vi "Cool Until Target.vi"(8 "error in (no error)":errorcluster, 10 "target temperature":dbl[unit]=273.15, 11 "cooling system in":refnum<class "Cooling System.lvclass">) -> (0 "error out":errorcluster, 3 "cooling system out":refnum<class "Cooling System.lvclass">)   [LabVIEW 2023, in "Cooling System.lvclass"]
uses:
  Cooling System.lvclass
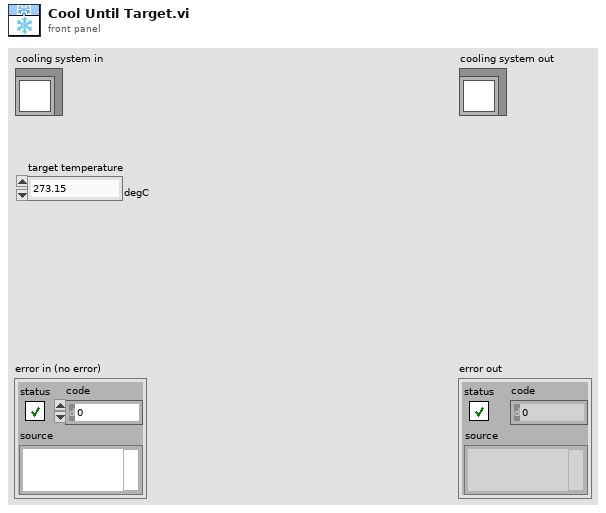
[diagram p1: front panel]
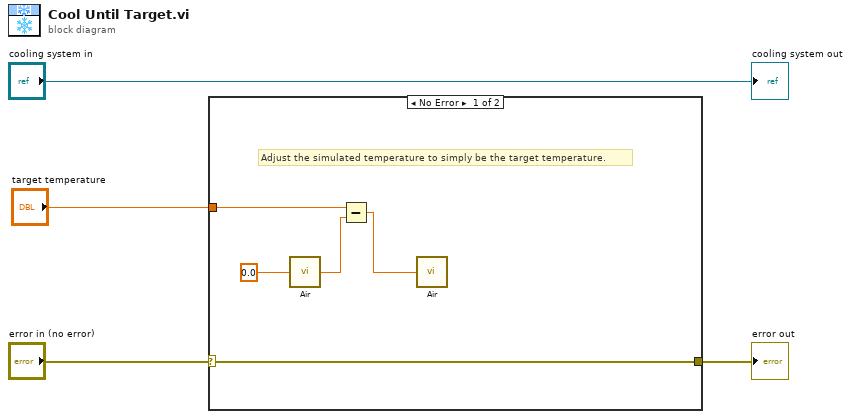
[diagram p0: block diagram]
diagram:
  n1 = case shown="No Error" "error in (no error)" {
    selector: "error in (no error)" -> [w5 w10]
    tunnel: "target temperature" -> [w7 _]
    tunnel: [w5 w10] -> w1
    frame No Error {
      # "Adjust the simulated temperature to simply be the target temperature."
      n2 = call "Air.vi"("temperature adjustment"=dbl[unit] 0.0) -> ("new air temperature"=w8:dbl[unit])
      n3 = Subtract(x=w7, y=w8) -> (x-y=w6:dbl[unit])
      n4 = call "Air.vi"("temperature adjustment"=w6) -> ()  [unwired: 1 out]
    }
    frame Error {
    }
  }
  "error out" <- w1
  "cooling system out" <- "cooling system in"
